vi "hw_triggering.vi"() -> ()   [LabVIEW 2021]
uses:
  <vilib>/userDefined/High Color/IMAQdx.ctl
  <vilib>/DAQmx/read.llb/DAQmx Read (Digital Bool 1Line 1Point).vi
  <vilib>/DAQmx/create/channels.llb/DAQmx Create Channel (DI-Digital Input).vi
  <vilib>/DAQmx/miscellaneous.llb/DAQmx Fill In Error Info.vi
  <vilib>/vision/driver/NI_Vision_Acquisition_Software.lvlib
panel:
  out "Trigger":bool
  in  "Slider":i32(slide)=3 max=9 scale=0.0..9.0
  in  "Stop analysis":bool
  out "Image":T1(plugin-control)
  in  "Frames":i32=10
  in  "VideoMode":u32=10
  in  "Session In":T2="cam0"
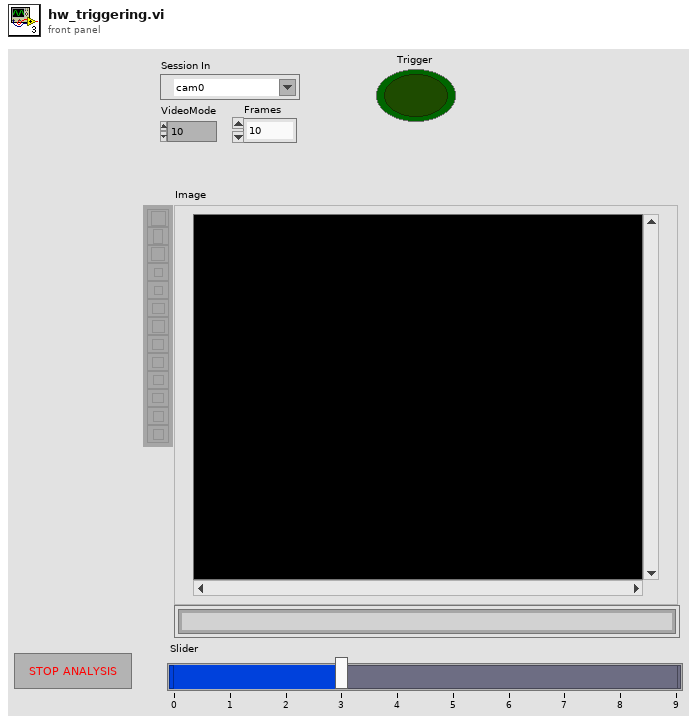
[diagram p1: front panel]
types:
  T1 = typedef "IMAQ Image.ctl" = refnum<image>
  T2 = typedef "IMAQdx.ctl" = refnum<k21>
  T3 = typedef "IMAQ AVI2 Refnum.ctl" = refnum<k20>
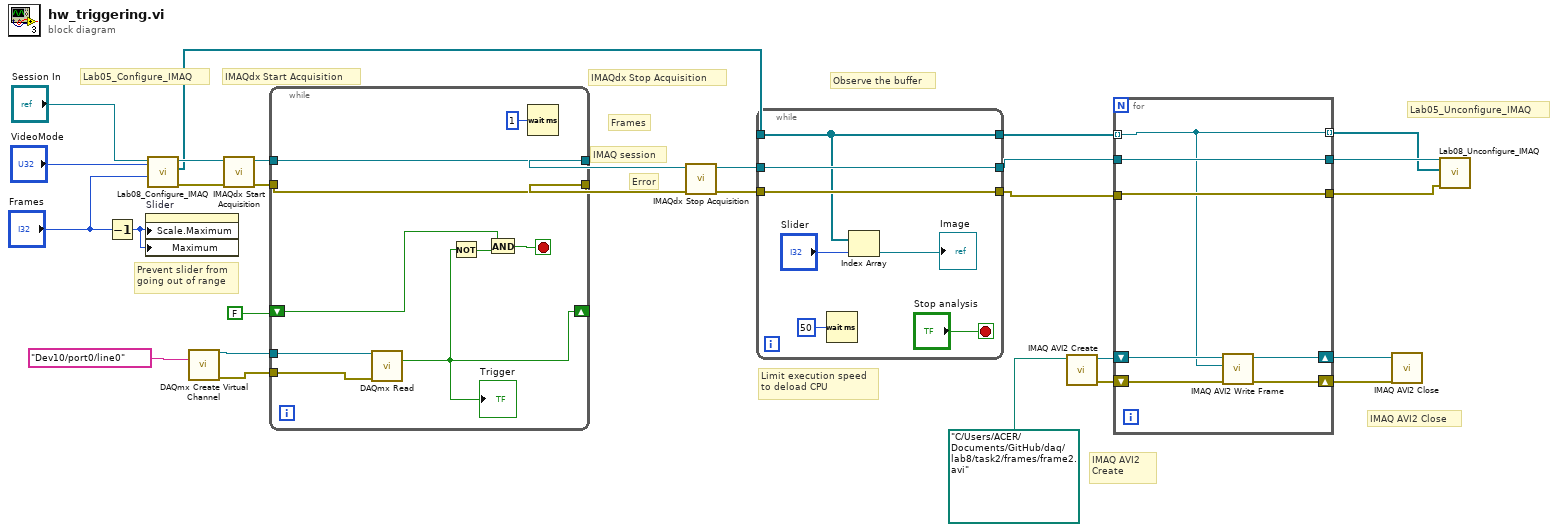
[diagram p0: block diagram]
diagram:
  # "IMAQ AVI2 Create"
  # "IMAQ AVI2 Close"
  # "Limit execution speed\nto deload CPU"
  # "Error"
  # "IMAQ session"
  # "Frames"
  # "Observe the buffer"
  # "Prevent slider from\ngoing out of range"
  # "Lab05_Unconfigure_IMAQ"
  # "Lab05_Configure_IMAQ"
  # "IMAQdx Stop Acquisition"
  # "IMAQdx Start Acquisition"
  n1 = Decrement(x="Frames") -> (x-1=w19:i32)
  n2 = property on="Slider" class="Slide (strict)"("Scale.Maximum"=w19, "Maximum"=w19) -> ()  [unwired: 2 in, 2 out]
  n3 = call "Lab08_Configure_IMAQ.vi"("Frames"="Frames", "VideoMode"="VideoMode", "Session In"="Session In") -> ("error out"=w25:errorcluster, "Images Out"=w18:T1[], "Session Out"=w26:T2)  [unwired: 2 in]
  n4 = call-poly <vilib>:"DAQmx Create Virtual Channel.vi"("lines"=tag "Dev10/port0/line0") -> ("task out"=w4:refnum<k21>, "error out"=w3:errorcluster)  [unwired: 13 in]
  n5 = call <vilib>:"IMAQdx Start Acquisition.vi"("error in"=w25, "Session In"=w26) -> ("error out"=w23:errorcluster, "Session Out"=w24:T2)  [unwired: 8 out]
  n6 = while {
    tunnel: w24 -> [w36]
    tunnel: w23 -> [w37]
    tunnel: [w37] -> w22
    tunnel: [w36] -> w21
    tunnel: w4 -> [w34]
    tunnel: w3 -> [w33]
    shift-right: [w30] -> _
    shift-left: FALSE ("data") -> [w29]
    stop <- w32 stop-if-true
    n7 = call-poly <vilib>:"DAQmx Read.vi"("task/channels in"=w34, "error in"=w33) -> ("data"=w30:bool)  [unwired: 11 in, 2 out]
    "Trigger" <- w30
    n8 = Not(x=w30) -> (.not. x?=w31:bool)
    n9 = And(x=w29, y=w31) -> (x .and. y?=w32:bool)
    n10 = Wait (ms)(milliseconds to wait=u32 1) -> ()  [unwired: 1 out]
  }
  n11 = call <vilib>:"IMAQdx Stop Acquisition.vi"("error in"=w22, "Session In"=w21) -> ("error out"=w16:errorcluster, "Session Out"=w17:T2)  [unwired: 8 out]
  n12 = while {
    tunnel: w18 -> [w39]
    tunnel: [w39] -> w8
    tunnel: w17 -> [w41]
    tunnel: [w41] -> w9
    tunnel: w16 -> [w40]
    tunnel: [w40] -> w10
    stop <- "Stop analysis" stop-if-true
    n13 = Wait (ms)(milliseconds to wait=u32 50) -> ()  [unwired: 1 out]
    n14 = Index Array "Index Array"(array=w39, index="Slider") -> (element=→"Image":T1)
  }
  n15 = call "IMAQ AVI2 Create"("AVI Path"=path "C:/Users/ACER/Documents/GitHub/daq/lab8/task2/frames/frame2.avi") -> ("error out"=w13:errorcluster, "AVI Refnum"=w12:T3)  [unwired: 9 in]
  n16 = for {
    shift-right: [w51] -> w15
    shift-left: w12 -> [w48]
    shift-right: [w50] -> w14
    shift-left: w13 -> [w49]
    tunnel: w10 -> [w47]
    tunnel: w9 -> [w46]
    tunnel: w8 -> [w45] mode=indexing
    tunnel: [w47] -> w7
    tunnel: [w46] -> w6
    tunnel: [w45] -> w5 mode=indexing
    n17 = call "IMAQ AVI2 Write Frame"("error in (no error)"=w49, "Image"=w45, "AVI Refnum"=w48) -> ("error out"=w50:errorcluster, "AVI Refnum (duplicate)"=w51:T3)  [unwired: 6 in, 1 out]
  }
  n18 = call "IMAQ AVI2 Close"("error in (no error)"=w14, "AVI Refnum"=w15) -> ()  [unwired: 9 in, 1 out]
  n19 = call "Lab08_Unconfigure_IMAQ.vi"("error in (no error)"=w7, "Images to dispose"=w5, "IMAQdx session in"=w6) -> ()  [unwired: 8 in, 1 out]
